vi "GetOverlay.vi"(8 "error in":errorcluster, 11 "Abstrace Instrument in":refnum<class "Abstract Instrument.lvclass">) -> (0 "error out":errorcluster, 2 "overlay":string, 3 "Abstract Instrument out":refnum<class "Abstract Instrument.lvclass">)   [LabVIEW 2025, in "Abstract Engine.lvlib" / "Abstract Instrument.lvclass"]
doc: "Copyright 2017 National Instruments Corporation\n\nLicensed under the Apache License, Version 2.0 (the \"License\"); you may not use this file except in compliance with the License. You may obtain a copy of the License at http://www.apache.org/licenses/LICENSE-2.0\nUnless required by applicable law or agreed to in writing, software distributed under the License is distributed on an \"AS IS\" BASIS, WITHOUT WARRANTIES OR CONDITIONS OF ANY KIND, either express or implied. See the License for the specific language governing permissions and limitations under the License."
uses:
  Abstract Instrument.lvclass
  Abstract Instrument.lvclass/Abstract Instrument.ctl
  Read error cluster.vi
  Users/Public/Documents/Sandia National Labs/TSS Plugin/CEF.lvlibp/serializable node/CEF_serializable node.lvclass
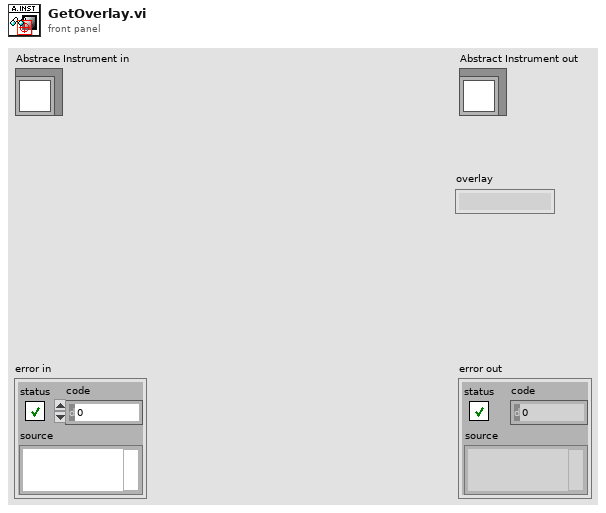
[diagram p1: front panel]
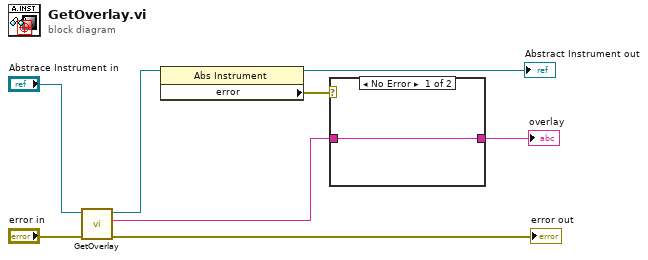
[diagram p0: block diagram]
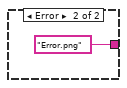
[diagram p2: hidden frame]
diagram:
  n1 = call-parent "GetOverlay.vi"("error in"="error in", "CEF_serializable node in"="Abstrace Instrument in") -> ("error out"=→"error out":errorcluster, "overlay"=w2:string, "CEF_serializable node out"=w6:refnum<class "Abstract Instrument.lvclass">)  [unwired: 7 in]
  n2 = property class="Abs Instrument"(reference=w6) -> (reference out=→"Abstract Instrument out":refnum<class "Abstract Instrument.lvclass">, "error"=w3:errorcluster)  [unwired: 1 in, 1 out]
  n3 = case shown="No Error" w3 {
    tunnel: w2 -> [w9 _]
    tunnel: [w9 "Error.png" ("overlay")] -> w1
    frame No Error {
    }
    frame Error {
    }
  }
  "overlay" <- w1
